vi "dbsys_save_logout.vi"() -> (1 "Статус":i32, 2 "Выход":i32)   [LabVIEW 2017]
uses:
  DBSysCore.dll
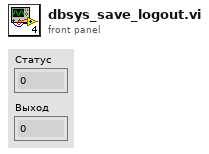
[diagram p1: front panel]
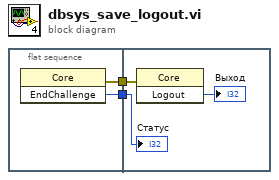
[diagram p0: block diagram]
diagram:
  n1 = flat-sequence {
    tunnel: [w4] -> w2
    tunnel: [w3] -> w1
    tunnel: w2 -> [w7]
    tunnel: w1 -> [w6]
    frame #0 {
      n2 = invoke class="Core" method="EndChallenge"() -> (error out=w4:errorcluster, "EndChallenge"=w3:i32)  [unwired: 3 in, 1 out]
    }
    frame #1 {
      n3 = invoke class="Core" method="Logout"(error in=w7) -> ("Logout"=→"Выход":i32)  [unwired: 2 in, 2 out]
      "Статус" <- w6
    }
  }
